vi "ChangeViPropExec.vi"() -> ()   [LabVIEW 2016]
panel:
  out "Slide":u8(slide) max=20 scale=0.0..31.0
  in  "Folder Path":path
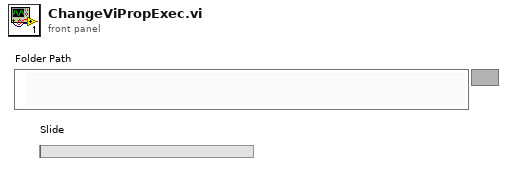
[diagram p1: front panel]
types:
  T1 = enum32{"invalid priority", "background priority", "normal priority", "above normal priority", "high priority", "time critical priority", "subroutine"}
  T2 = enum16{"Share clones between instances", "Preallocate clone for each instance"}
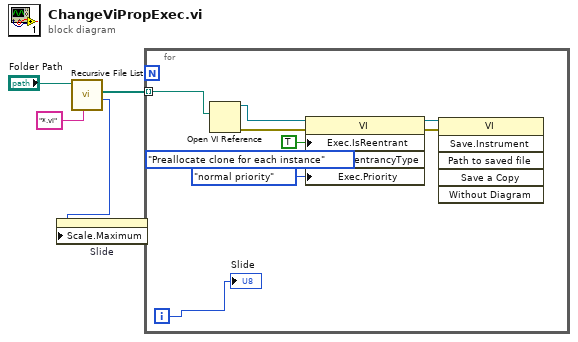
[diagram p0: block diagram]
diagram:
  n1 = call <vilib>:"Recursive File List.vi"("pattern"="*.vi", "Folder Path"="Folder Path") -> ("Number of Files"=w1:i32, "All Files in Dir"=w2:path[])  [unwired: 5 in, 3 out]
  n2 = property on="Slide" class="Slide (strict)"("Scale.Maximum"=w1) -> ()  [unwired: 2 in, 2 out]
  n3 = for {
    tunnel: w2 -> [w13] mode=indexing
    i -> [w5]
    n4 = Open VI Reference(vi path=w13) -> (vi reference=w12:refnum<vi>, error out=w11:errorcluster)  [unwired: 5 in]
    n5 = property class="VI"(reference=w12, error in=w11, "Exec.IsReentrant"=TRUE ("Execution:Is Reentrant"), "Exec.ReentrancyType"=T2."Preallocate clone for each instance" ("Execution:Reentrancy Type"), "Exec.Priority"=T1."normal priority" ("Execution:Priority")) -> (reference out=w7:refnum<vi>, error out=w6:errorcluster)
    n6 = invoke class="VI" method="Save.Instrument"(reference=w7, error in=w6) -> ()  [unwired: 4 in, 6 out]
    "Slide" <- w5
  }
